vi "ArrayElementBG.vi"(8 "error in":errorcluster, 11 "Arr Refnum":refnum<vi>) -> (0 "error out":errorcluster, 3 "Arr Refnum out":refnum<vi>, 5 "Element BG":u32(colorbox))   [LabVIEW 2014, in "Array.lvclass"]
uses:
  Array.lvclass
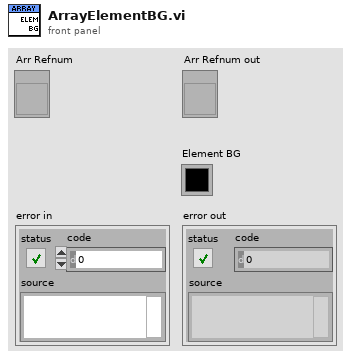
[diagram p1: front panel]
types:
  T1 = typedef "LVRectTypeDef.ctl" = cluster{"Left":i16, "Top":i16, "Right":i16, "Bottom":i16}
  T2 = typedef "LVPositionTypeDef.ctl" = cluster{"Left":i32, "Top":i32}
  T3 = typedef "imagedata.ctl" = cluster{"image type":i32, "image depth":i32, "image":u8[], "mask":u8[], "colors":u32[], "Rectangle":cluster{"left":i16, "top":i16, "right":i16, "bottom":i16}}
  T4 = cluster{"left":i16, "top":i16, "right":i16, "bottom":i16}
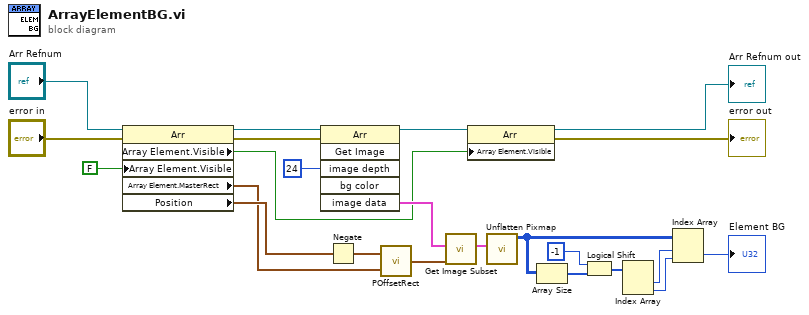
[diagram p0: block diagram]
diagram:
  n1 = property on="Property Node" class="Arr"(reference="Arr Refnum", error in="error in", "Array Element.Visible"=FALSE) -> (reference out=w7:refnum<vi>, error out=w22:errorcluster, "Array Element.Visible"=w1:bool, "Array Element.MasterRect"=w17:T1, "Position"=w19:T2)
  n2 = invoke on="Invoke Node" class="Arr" method="Get Image"(reference=w7, error in=w22, "image depth"=24 ("Image Depth")) -> (reference out=w4:refnum<vi>, "image data"=w20:T3)  [unwired: 3 in, 4 out]
  n3 = Negate(x=w19) -> (-x=w16:T2)
  n4 = call <vilib>:"POffsetRect.vi"("rect"=w17, "point"=w16) -> ("offset rect"=w18:T4)
  n5 = call <vilib>:"Get Image Subset.vi"("subset rect"=w18, "image data"=w20) -> ("image subset"=w15:T3)  [unwired: 4 in, 1 out]
  n6 = property on="Property Node" class="Arr"(reference=w4, "Array Element.Visible"=w1) -> (reference out=→"Arr Refnum out":refnum<vi>, error out=→"error out":errorcluster)  [unwired: 1 in]
  n7 = call <vilib>:"Unflatten Pixmap.vi"("image data"=w15) -> ("24-bit pixmap"=w11:u32[][])  [unwired: 4 in, 6 out]
  n8 = Array Size(array=w11) -> (size(s)=w12:i32[])
  n9 = Logical Shift(y=i16 -1, x=w12) -> (x << y=w10:i32[])
  n10 = Index Array(array=w10) -> (element #1=w9:i32, element #2=w8:i32)  [unwired: 2 in]
  n11 = Index Array(array=w11, index (row)=w9, index (col)=w8) -> (element=→"Element BG":u32)
